vi "Truncate String.vi"(9 "direction":enum16{"Front", "Back"}(ring)=enum."Back", 10 "# of characters to remove":u32, 11 "string":string) -> (2 "removed all?":bool, 3 "truncated string":string)   [LabVIEW 2024, in "Logging.lvlib" / "Format String.lvclass"]
uses:
  Format String.lvclass
panel:
  # "Connector Pane"
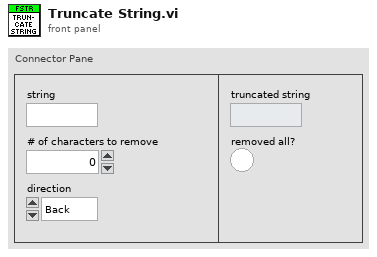
[diagram p1: front panel]
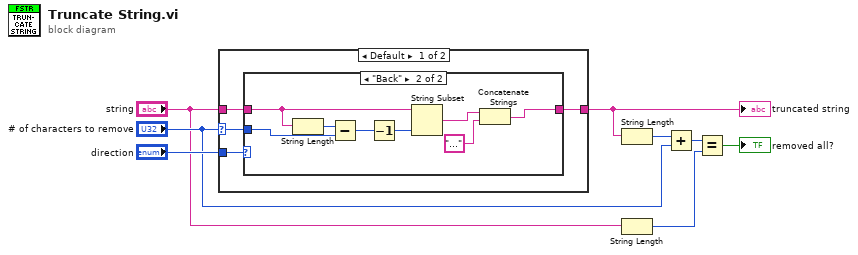
[diagram p0: block diagram]
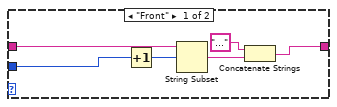
[diagram p2: hidden frame]
diagram:
  n1 = case shown="Default" "# of characters to remove" {
    selector: "# of characters to remove" -> [w11 _]
    tunnel: [w12 w27] -> w7
    tunnel: "string" -> [w10 w27]
    tunnel: "direction" -> [w9 _]
    frame Default {
      n2 = case shown="\"Back\"" w9 {
        tunnel: [w18 w26] -> w12
        tunnel: w11 -> [w15 w23]
        tunnel: w10 -> [w14 w25]
        frame "Front" {
          n3 = Increment(x=w15) -> (x+1=w13:u32)
          n4 = String Subset(string=w14, offset (0)=w13) -> (substring=w16:string)  [unwired: 1 in]
          n5 = Concatenate Strings("…", w16) -> (w18:string)
        }
        frame "Back" {
          n6 = String Length(string=w25) -> (length=w24:i32)
          n7 = Subtract(x=w24, y=w23) -> (x-y=w22:u32)
          n8 = Decrement(x=w22) -> (x-1=w19:u32)
          n9 = String Subset(string=w25, length (rest)=w19) -> (substring=w20:string)  [unwired: 1 in]
          n10 = Concatenate Strings(w20, "…") -> (w26:string)
        }
      }
    }
    frame 0 {
    }
  }
  "truncated string" <- w7
  n11 = String Length(string=w7) -> (length=w6:i32)
  n12 = String Length(string="string") -> (length=w2:i32)
  n13 = Add(x=w6, y="# of characters to remove") -> (x+y=w3:u32)
  n14 = Equal?(x=w3, y=w2) -> (x = y?=→"removed all?":bool)
